vi "I2C Operation.vi"(6 "input_data":u8[](array[numeric])=[255, 255, 255, 255] format="%.0x", 7 "size":i32, 8 "Channel":u8 max=5 step=1, 9 "address":u8=123, 10 "mode":string(combo)="write", 11 "VISA":refnum<visa-resource-name>="COM3") -> (0 "VISA  2":refnum<visa-resource-name>="COM3", 1 "result":bool, 2 "message":string="no match!", 3 "Data Out":u8[](array[numeric]) format="%.0x")   [LabVIEW 2011]
panel:
  in  "write_delay":dbl=250.0
  in  "read_delay":dbl=0.1
  out "无符号字节数组":u8[](array[numeric])=[238, 0, 13, 4, 0, 161, 0, 0, 3, 4, 33, 1, 0, 0, 0, 65, 132, 128, 85, 0, 103, 0, 0, 0, 0, 0, 5, 0, 68, 69, 76, 76, 32, 32, 32, 32, 32, 32, 32, 32, 32, 32, 32, 32, 0, 60, 24, 160, 76, 53, 54, 81, 70, 48, 51, 48, 45, 83, 68, 45, 82, 32, 32, 32, 66, 32, 32, 32, 1, 0, 0, 235, 0, 0, 0, 0, 49, 54, 48, 50, 56, 48, 48, 50, 56, 32, 32, 32, 32, 32, 32, 32, 49, 54, 48, 49, 50, 56, 32, 32, 0, 0, 0, 29, 15, 16, 0, 163, 132, 0, 0, 255, 255, 255, 255, 255, 255, 255, 255, 255, 255, 255, 255, 255, 255, 255, 255, 255, 255, 255, 255, 255, 255, 255, 255, 255, 255, 255, 255, 255, 255, 255, 255, 255, 255, 255, 255, 255, 255, 255, 255, 255, 255, 255, 255, 255, 255, 255, 255, 255, 255, 255, 255, 255, 255, 255, 255, 255, 255, 255, 255, 255, 255, 255, 255, 255, 255, 255, 255, 255, 255, 255, 255, 255, 255, 255, 255, 255, 255, 255, 255, 255, 255, 255, 255, 255, 255, 255, 255, 255, 255, 255, 255, 255, 255, 255, 255, 255, 255, 255, 255, 255, 255, 255, 255, 255, 255, 255, 255, 255, 255, 255, 255, 255, 255, 255, 255, 255, 255, 255, 255, 255, 255, 255, 255, 255, 255, 255, 255, 255, 255, 255, 255, 255, 255, 255, 255, 255, 255, 255, 255, 255, 255, 255, 255, 255, 255, 255, 255, 255, 255, 255, 255, 255, 63, 255, 252, 255, 255] format="%.0x"
  out "write error":string
  out "read error":u8[](array[numeric]) format="%.0x"
  # "0"
  # "1"
  # "2"
  # "3"
  # "4"
  # "5"
  # "6"
  # "7"
  # "8"
  # "9"
  # "10"
  # "11"
  # "12"
  # "13"
  # "14"
  # "15"
  # "16"
  # "17"
  # "18"
  # "19"
  # "20"
  # "21"
  # "I2C EEPROM Opertion"
  # "10"
  # "0"
  # "5"
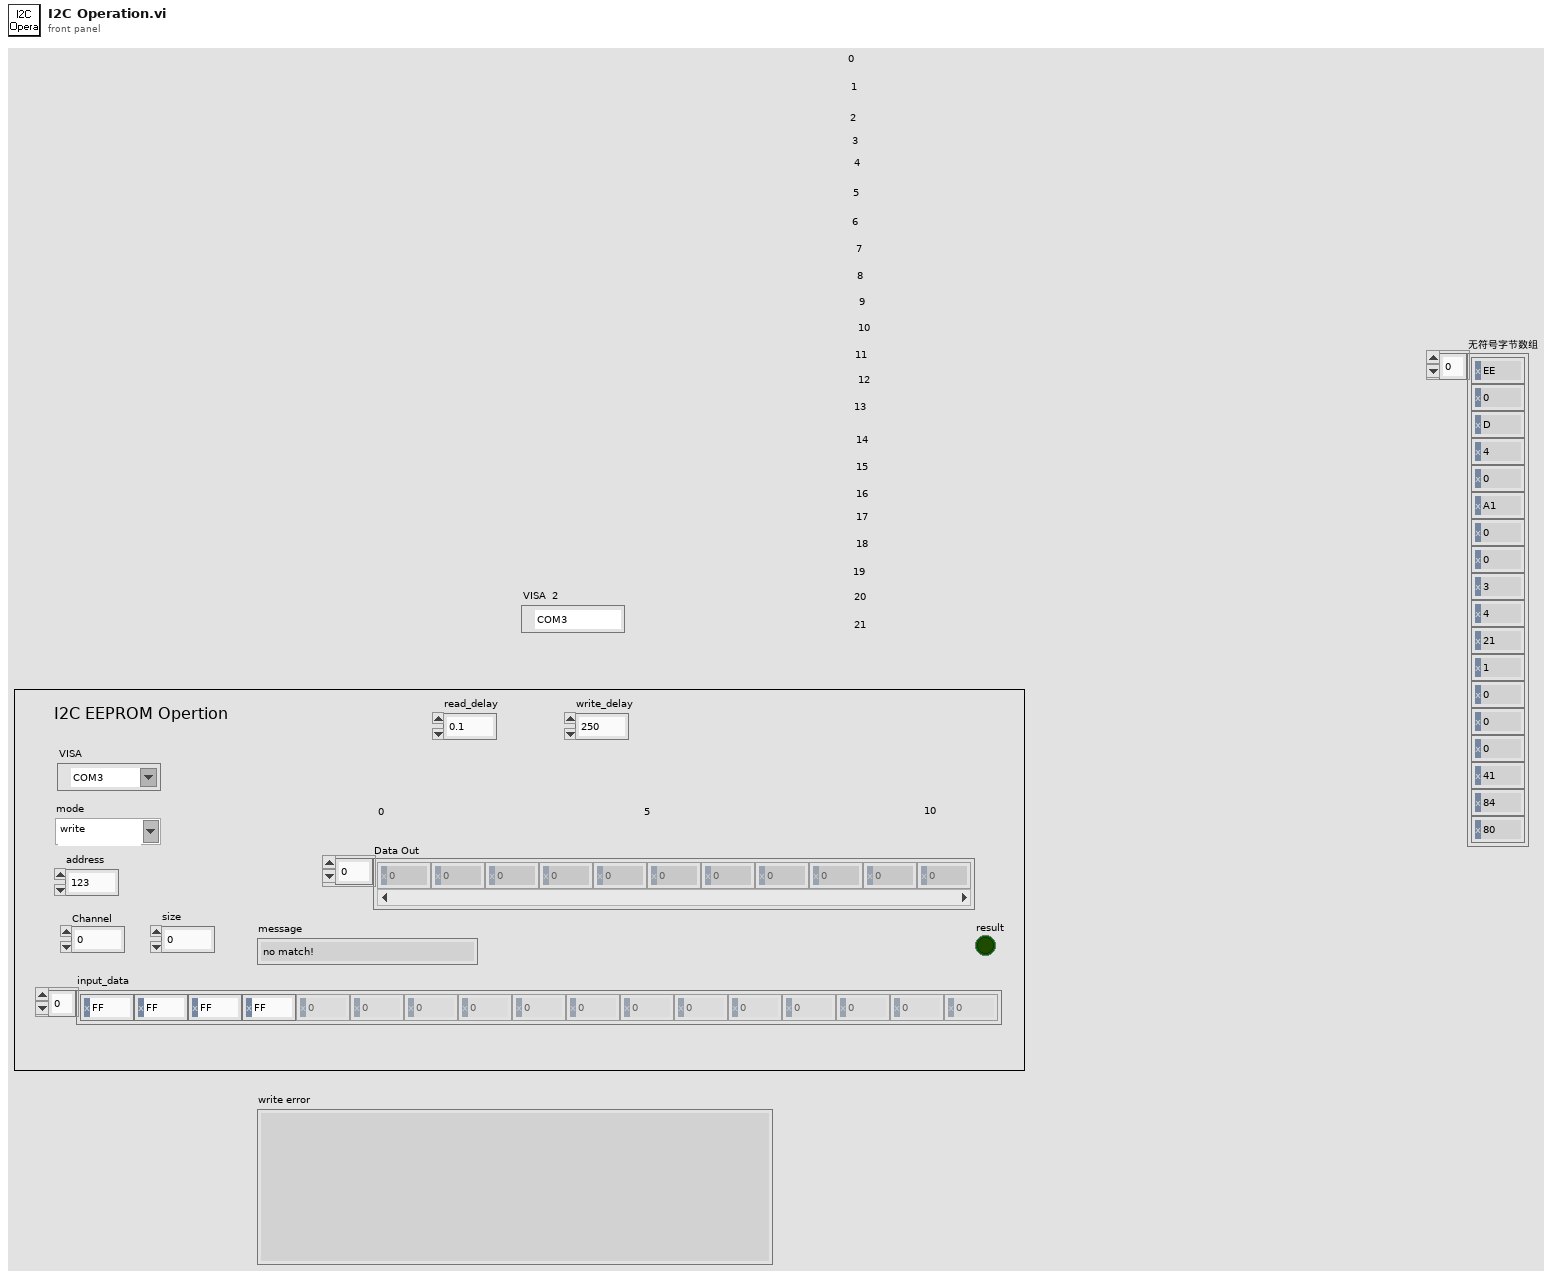
[diagram p1: front panel]
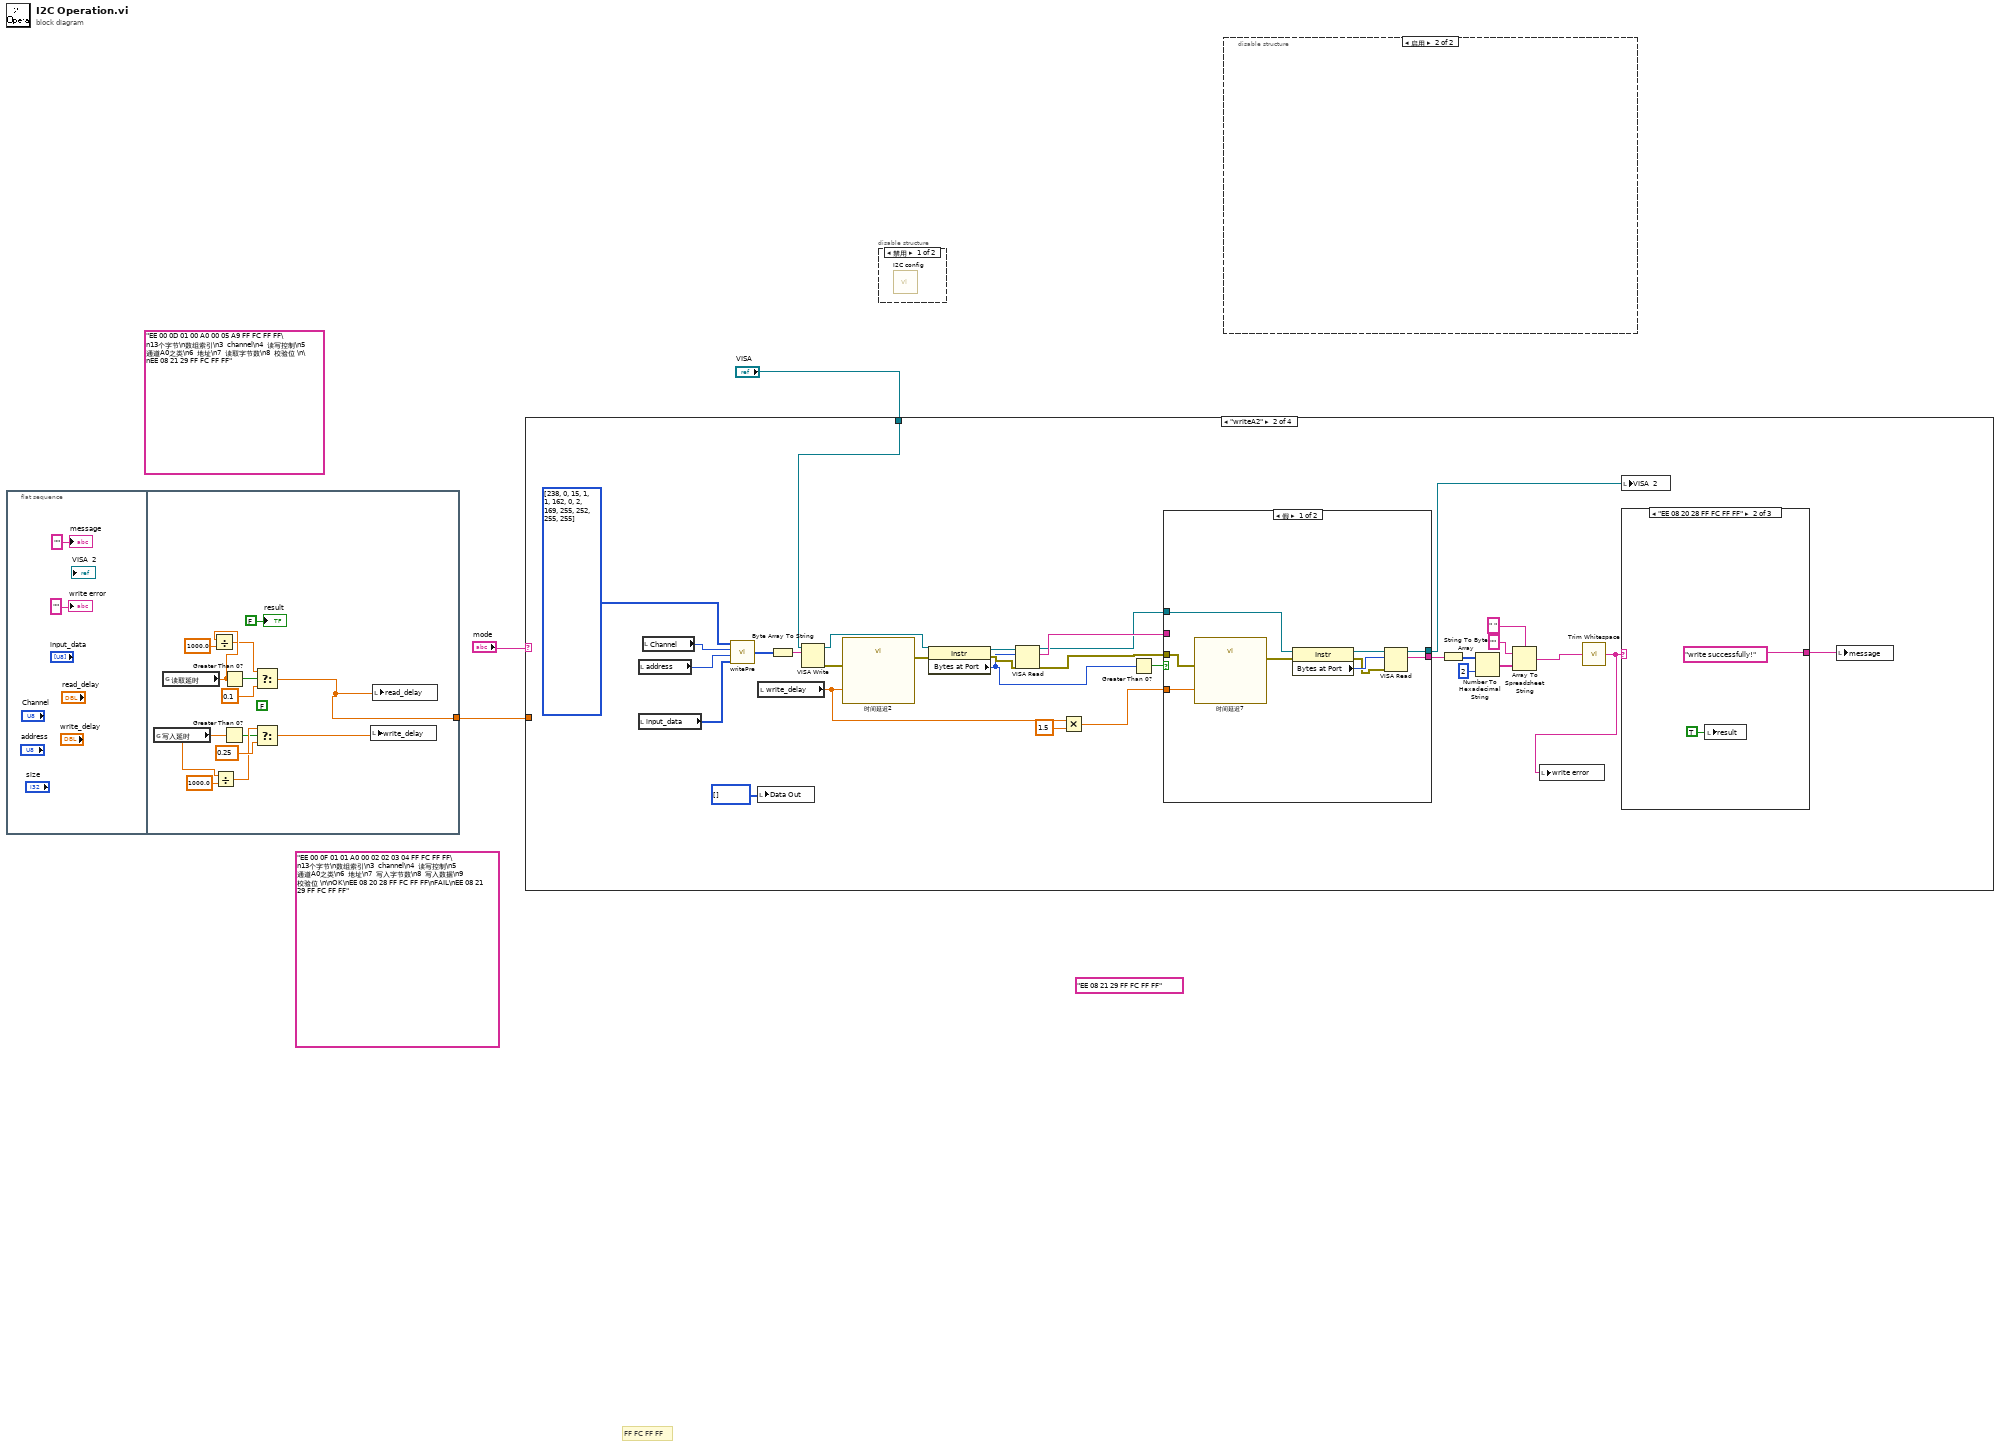
[diagram p0: block diagram]
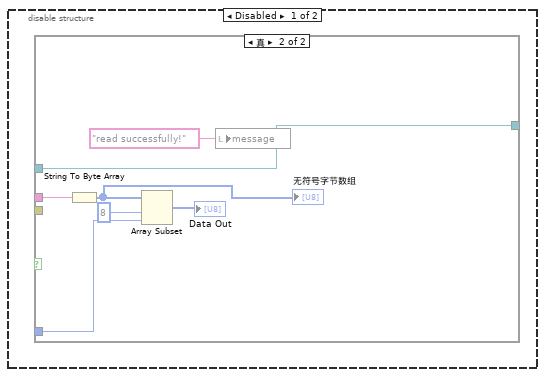
[diagram p2: hidden frame]
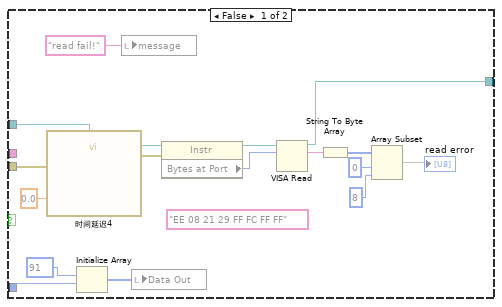
[diagram p3: hidden frame]
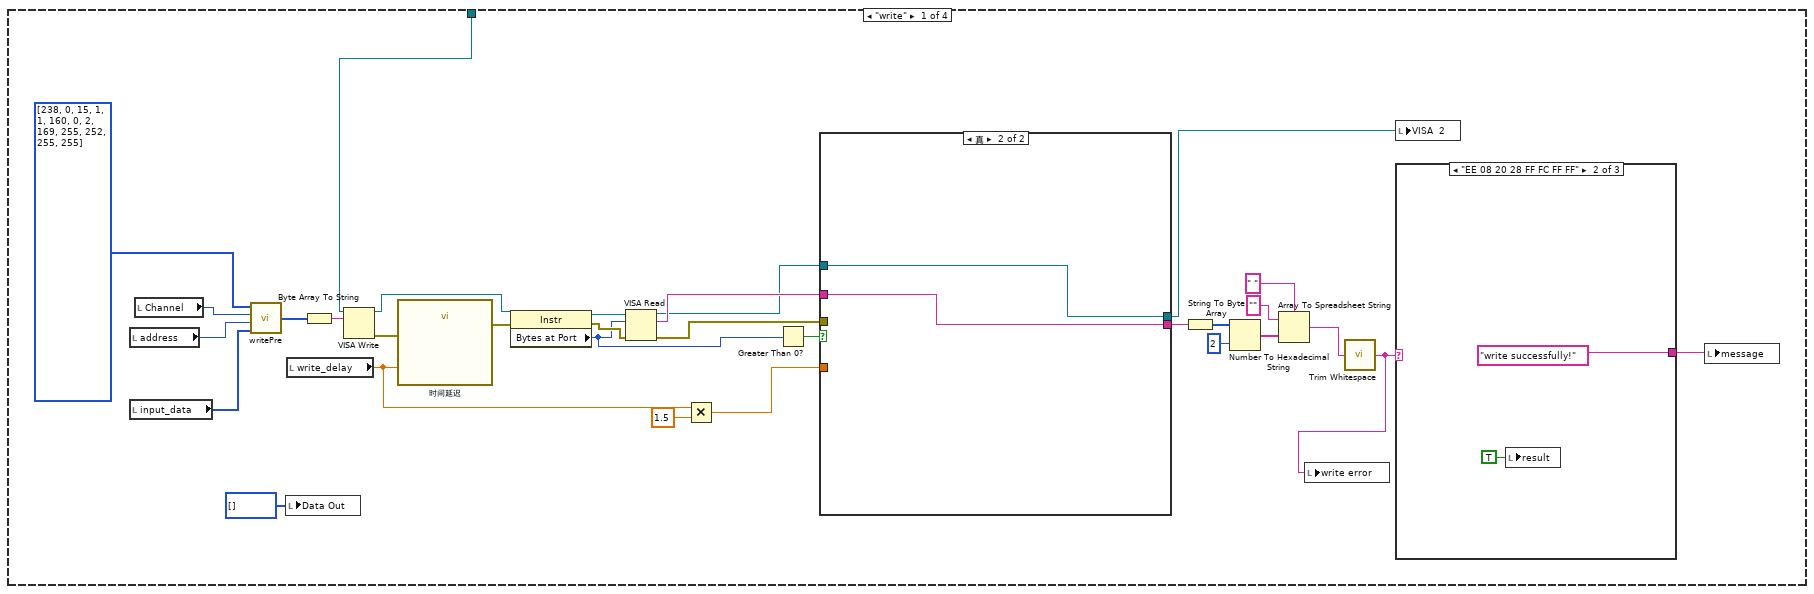
[diagram p5: hidden frame]
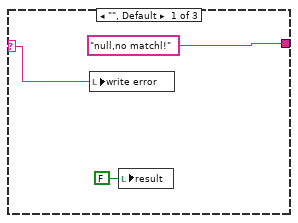
[diagram p6: hidden frame]
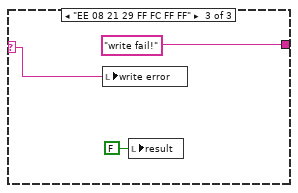
[diagram p7: hidden frame]
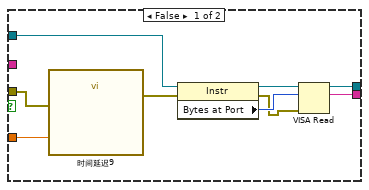
[diagram p8: hidden frame]
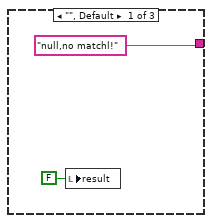
[diagram p9: hidden frame]
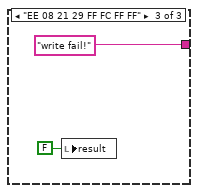
[diagram p10: hidden frame]
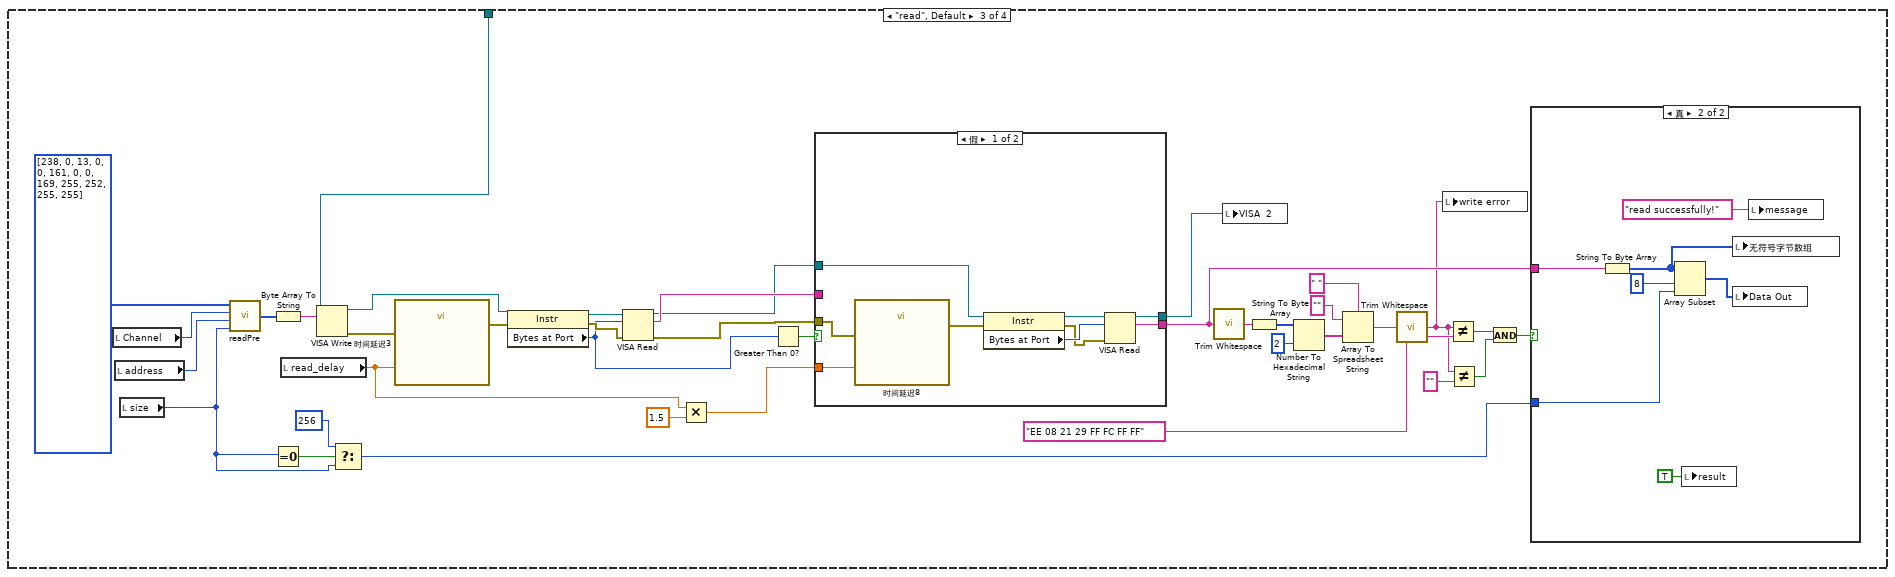
[diagram p12: hidden frame]
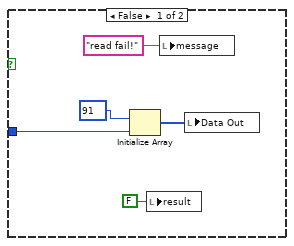
[diagram p13: hidden frame]
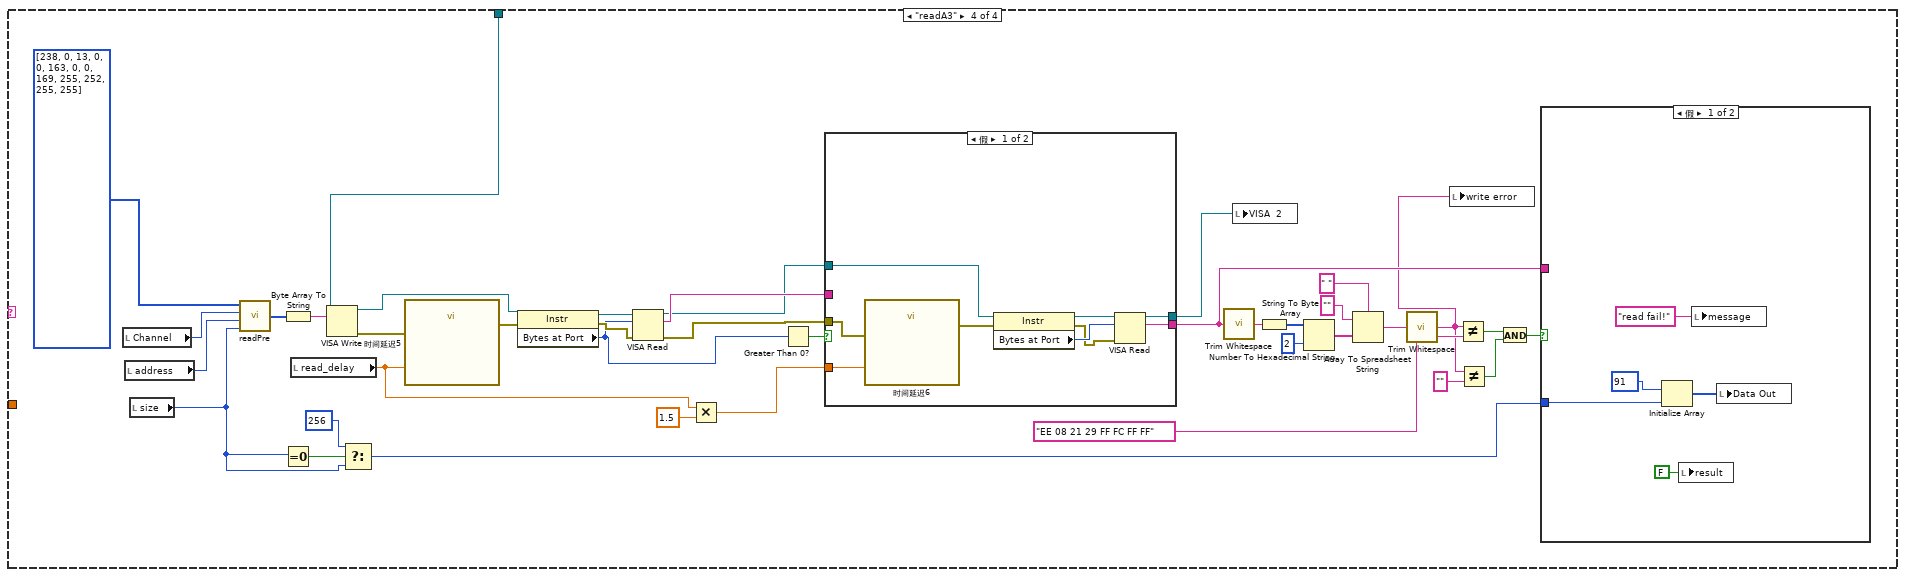
[diagram p15: hidden frame]
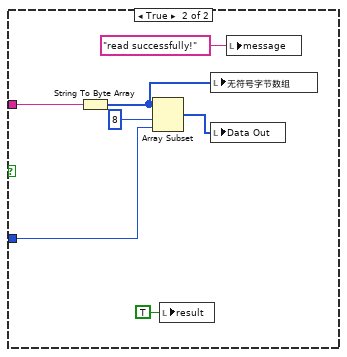
[diagram p16: hidden frame]
diagram:
  (unwired) "EE 08 21 29 FF FC FF FF"
  (unwired) "EE 00 0F 01 01 A0 00 02 02 03 04 FF FC FF FF\n13个字节\n数组索引\n3  channel\n4  读写控制\n5  通道A0之类\n6  地址\n7  写入字节数\n8  写入数据\n9  校验位 \n\nOK\nEE 08 20 28 FF FC FF FF\nFAIL\nEE 08 21 29 FF FC FF FF"
  (unwired) "EE 00 0D 01 00 A0 00 05 A9 FF FC FF FF\n13个字节\n数组索引\n3  channel\n4  读写控制\n5  通道A0之类\n6  地址\n7  读取字节数\n8  校验位 \n\nEE 08 21 29 FF FC FF FF"
  # "FF FC FF FF"
  n1 = flat-sequence {
    tunnel: [w10] -> w2
    frame #0 {
      "write error" <- "" ("write error")
      "message" <- "" ("message")
    }
    frame #1 {
      (unwired) FALSE ("s")
      n2 = global read "延时设置全局变量.vi" "写入延时"() -> (w8:dbl)
      n3 = global read "延时设置全局变量.vi" "读取延时"() -> (w12:dbl)
      n4 = Divide(x=w12, y=1000.0) -> (x/y=w11:dbl)
      n5 = Divide(x=w8, y=1000.0) -> (x/y=w9:dbl)
      n6 = Greater Than 0?(x=w8) -> (x > 0?=w6:bool)
      n7 = Greater Than 0?(x=w12) -> (x > 0?=w15:bool)
      n8 = Select(t=w9, s=w6, f=0.25) -> (s? t:f=w7:dbl)
      n9 = Select(t=w11, s=w15, f=0.1) -> (s? t:f=w10:dbl)
      n10 = local write "write_delay"(w7) -> ()
      n11 = local write "read_delay"(w10) -> ()
      "result" <- FALSE ("result")
    }
  }
  n12 = case shown="\"writeA2\"" "mode" {
    tunnel: "VISA" -> [w38 w89 w152 w213]
    tunnel: w2 -> [_ _ _ _]
    frame "write" {
      n13 = local read "address"() -> (w44:u8)
      n14 = local read "input_data"() -> (w23:u8[])
      n15 = local read "Channel"() -> (w45:u8)
      n16 = call "writePre.vi"("input_data"=w23, "address"=w44, "Channel"=w45, "order"=u8[] [238, 0, 15, 1, 1, 160, 0, 2, 169, 255, 252, 255, 255]) -> ("out"=w42:u8[])
      n17 = local write "Data Out"(u8[] [] ("Data Out")) -> ()
      n18 = local read "write_delay"() -> (w36:dbl)
      n19 = Byte Array To String(unsigned byte array=w42) -> (string=w49:string)
      n20 = VISA Write(VISA resource name=w38, write buffer=w49) -> (VISA resource name out=w39:refnum<visa-resource-name>, error out=w40:errorcluster)  [unwired: 1 in, 1 out]
      n21 = call "时间延迟"("error in (no error)"=w40, "Delay Time (s)"=w36) -> ("error out"=w47:errorcluster)  [unwired: 9 in]
      n22 = property class="Instr"(reference=w39, error in=w47) -> (reference out=w48:refnum<visa-resource-name>, error out=w46:errorcluster, "Bytes at Port"=w22:u32)
      n23 = VISA Read(VISA resource name=w48, byte count=w22, error in (no error)=w46) -> (VISA resource name out=w21:refnum<visa-resource-name>, read buffer=w26:string, error out=w20:errorcluster)  [unwired: 1 out]
      n24 = Multiply(x=w36, y=1.5) -> (x*y=w34:dbl)
      n25 = Greater Than 0?(x=w22) -> (x > 0?=w37:bool)
      n26 = case shown="真" w37 {
        tunnel: w34 -> [w66 _]
        tunnel: w20 -> [w65 _]
        tunnel: w21 -> [w64 w67]
        tunnel: [w59 w68] -> w27
        tunnel: w26 -> [_ w68]
        tunnel: [w58 w67] -> w24
        frame False {
          n27 = call "时间延迟9"("error in (no error)"=w65, "Delay Time (s)"=w66) -> ("error out"=w63:errorcluster)  [unwired: 9 in]
          n28 = property class="Instr"(reference=w64, error in=w63) -> (reference out=w62:refnum<visa-resource-name>, error out=w60:errorcluster, "Bytes at Port"=w61:u32)
          n29 = VISA Read(VISA resource name=w62, byte count=w61, error in (no error)=w60) -> (VISA resource name out=w58:refnum<visa-resource-name>, read buffer=w59:string)  [unwired: 2 out]
        }
        frame True {
        }
      }
      n30 = String To Byte Array(string=w27) -> (unsigned byte array=w33:u8[])
      n31 = Number To Hexadecimal String(1:i16 2 ("宽度(-)"), 2:w33) -> (0:w32:string[])
      n32 = Array To Spreadsheet String(delimiter (Tab)=" " ("分隔符(Tab)"), array=w32, 3:"" ("格式字符串")) -> (spreadsheet string=w29:string)
      n33 = call <vilib>:"Trim Whitespace.vi"("string"=w29) -> ("trimmed string"=w19:string)  [unwired: 1 in]
      n34 = local write "write error"(w19) -> ()
      n35 = local write "VISA  2"(w24) -> ()
      n36 = case shown="\"EE 08 20 28 FF FC FF FF\"" w19 {
        selector: w19 -> [w50 _ w55]
        tunnel: ["null,no matchl!" "write successfully!" "write fail!"] -> w25
        frame "", Default {
          n37 = local write "write error"(w50) -> ()
          n38 = local write "result"(FALSE ("result")) -> ()
        }
        frame "EE 08 20 28 FF FC FF FF" {
          n39 = local write "result"(TRUE ("result")) -> ()
        }
        frame "EE 08 21 29 FF FC FF FF" {
          n40 = local write "write error"(w55) -> ()
          n41 = local write "result"(FALSE ("result")) -> ()
        }
      }
      n42 = local write "message"(w25) -> ()
    }
    frame "writeA2" {
      n43 = local read "address"() -> (w94:u8)
      n44 = local read "input_data"() -> (w74:u8[])
      n45 = local read "Channel"() -> (w95:u8)
      n46 = call "writePre.vi"("input_data"=w74, "address"=w94, "Channel"=w95, "order"=u8[] [238, 0, 15, 1, 1, 162, 0, 2, 169, 255, 252, 255, 255]) -> ("out"=w93:u8[])
      n47 = local write "Data Out"(u8[] [] ("Data Out")) -> ()
      n48 = local read "write_delay"() -> (w87:dbl)
      n49 = Byte Array To String(unsigned byte array=w93) -> (string=w99:string)
      n50 = VISA Write(VISA resource name=w89, write buffer=w99) -> (VISA resource name out=w90:refnum<visa-resource-name>, error out=w91:errorcluster)  [unwired: 1 in, 1 out]
      n51 = call "时间延迟2"("error in (no error)"=w91, "Delay Time (s)"=w87) -> ("error out"=w97:errorcluster)  [unwired: 9 in]
      n52 = property class="Instr"(reference=w90, error in=w97) -> (reference out=w98:refnum<visa-resource-name>, error out=w96:errorcluster, "Bytes at Port"=w70:u32)
      n53 = VISA Read(VISA resource name=w98, byte count=w70, error in (no error)=w96) -> (VISA resource name out=w72:refnum<visa-resource-name>, read buffer=w77:string, error out=w71:errorcluster)  [unwired: 1 out]
      n54 = Multiply(x=w87, y=1.5) -> (x*y=w85:dbl)
      n55 = Greater Than 0?(x=w70) -> (x > 0?=w88:bool)
      n56 = case shown="假" w88 {
        tunnel: w85 -> [w114 _]
        tunnel: w71 -> [w113 _]
        tunnel: w72 -> [w112 w115]
        tunnel: [w107 w116] -> w78
        tunnel: w77 -> [_ w116]
        tunnel: [w106 w115] -> w75
        frame False {
          n57 = call "时间延迟7"("error in (no error)"=w113, "Delay Time (s)"=w114) -> ("error out"=w111:errorcluster)  [unwired: 9 in]
          n58 = property class="Instr"(reference=w112, error in=w111) -> (reference out=w110:refnum<visa-resource-name>, error out=w108:errorcluster, "Bytes at Port"=w109:u32)
          n59 = VISA Read(VISA resource name=w110, byte count=w109, error in (no error)=w108) -> (VISA resource name out=w106:refnum<visa-resource-name>, read buffer=w107:string)  [unwired: 2 out]
        }
        frame True {
        }
      }
      n60 = String To Byte Array(string=w78) -> (unsigned byte array=w84:u8[])
      n61 = Number To Hexadecimal String(1:i16 2 ("宽度(-)"), 2:w84) -> (0:w83:string[])
      n62 = Array To Spreadsheet String(delimiter (Tab)=" " ("分隔符(Tab)"), array=w83, 3:"" ("格式字符串")) -> (spreadsheet string=w80:string)
      n63 = call <vilib>:"Trim Whitespace.vi"("string"=w80) -> ("trimmed string"=w69:string)  [unwired: 1 in]
      n64 = local write "write error"(w69) -> ()
      n65 = local write "VISA  2"(w75) -> ()
      n66 = case shown="\"EE 08 20 28 FF FC FF FF\"" w69 {
        tunnel: ["null,no matchl!" "write successfully!" "write fail!"] -> w76
        frame "", Default {
          n67 = local write "result"(FALSE ("result")) -> ()
        }
        frame "EE 08 20 28 FF FC FF FF" {
          n68 = local write "result"(TRUE ("result")) -> ()
        }
        frame "EE 08 21 29 FF FC FF FF" {
          n69 = local write "result"(FALSE ("result")) -> ()
        }
      }
      n70 = local write "message"(w76) -> ()
    }
    frame "read", Default {
      n71 = local read "Channel"() -> (w123:u8)
      n72 = local read "address"() -> (w122:u8)
      n73 = local read "size"() -> (w121:i32)
      n74 = call "readPre.vi"("size"=w121, "address"=w122, "Channel"=w123, "input_order"=u8[] [238, 0, 13, 0, 0, 161, 0, 0, 169, 255, 252, 255, 255]) -> ("out"=w148:u8[])
      n75 = Byte Array To String(unsigned byte array=w148) -> (string=w154:string)
      n76 = Equal To 0?(x=w121) -> (x = 0?=w147:bool)
      n77 = local read "read_delay"() -> (w139:dbl)
      n78 = VISA Write(VISA resource name=w152, write buffer=w154) -> (VISA resource name out=w145:refnum<visa-resource-name>, error out=w144:errorcluster)  [unwired: 1 in, 1 out]
      n79 = Select(t=256, s=w147, f=w121) -> (s? t:f=w131:i32)
      n80 = call "时间延迟3"("error in (no error)"=w144, "Delay Time (s)"=w139) -> ("error out"=w151:errorcluster)  [unwired: 9 in]
      n81 = property class="Instr"(reference=w145, error in=w151) -> (reference out=w153:refnum<visa-resource-name>, error out=w150:errorcluster, "Bytes at Port"=w118:u32)
      n82 = VISA Read(VISA resource name=w153, byte count=w118, error in (no error)=w150) -> (VISA resource name out=w120:refnum<visa-resource-name>, read buffer=w140:string, error out=w119:errorcluster)  [unwired: 1 out]
      n83 = Multiply(x=w139, y=1.5) -> (x*y=w141:dbl)
      n84 = Greater Than 0?(x=w118) -> (x > 0?=w143:bool)
      n85 = case shown="假" w143 {
        tunnel: w141 -> [w175 _]
        tunnel: w119 -> [w174 _]
        tunnel: w120 -> [w173 w176]
        tunnel: [w168 w177] -> w133
        tunnel: w140 -> [_ w177]
        tunnel: [w167 w176] -> w132
        frame False {
          n86 = call "时间延迟8"("error in (no error)"=w174, "Delay Time (s)"=w175) -> ("error out"=w172:errorcluster)  [unwired: 9 in]
          n87 = property class="Instr"(reference=w173, error in=w172) -> (reference out=w171:refnum<visa-resource-name>, error out=w169:errorcluster, "Bytes at Port"=w170:u32)
          n88 = VISA Read(VISA resource name=w171, byte count=w170, error in (no error)=w169) -> (VISA resource name out=w167:refnum<visa-resource-name>, read buffer=w168:string)  [unwired: 2 out]
        }
        frame True {
        }
      }
      n89 = call <vilib>:"Trim Whitespace.vi"("string"=w133) -> ("trimmed string"=w125:string)  [unwired: 1 in]
      n90 = local write "VISA  2"(w132) -> ()
      n91 = String To Byte Array(string=w125) -> (unsigned byte array=w130:u8[])
      n92 = Number To Hexadecimal String(1:i16 2 ("宽度(-)"), 2:w130) -> (0:w129:string[])
      n93 = Array To Spreadsheet String(delimiter (Tab)=" " ("分隔符(Tab)"), array=w129, 3:"" ("格式字符串")) -> (spreadsheet string=w124:string)
      n94 = call <vilib>:"Trim Whitespace.vi"("string"=w124) -> ("trimmed string"=w117:string)  [unwired: 1 in]
      n95 = local write "write error"(w117) -> ()
      n96 = Not Equal?(x=w117, y="EE 08 21 29 FF FC FF FF") -> (x != y?=w136:bool)
      n97 = Not Equal?(x=w117, y="") -> (x != y?=w135:bool)
      n98 = And(x=w136, y=w135) -> (x .and. y?=w134:bool)
      n99 = case shown="真" w134 {
        tunnel: w133 -> [_ w165]
        tunnel: w131 -> [w156 w163]
        frame False {
          n100 = Initialize Array(u8 91, w156) -> (w157:u8[])
          n101 = local write "result"(FALSE ("result")) -> ()
          n102 = local write "message"("read fail!" ("message")) -> ()
          n103 = local write "Data Out"(w157) -> ()
        }
        frame True {
          n104 = String To Byte Array(string=w165) -> (unsigned byte array=w162:u8[])
          n105 = Array Subset(array=w162, index=8 ("索引"), length=w163) -> (w161:u8[])
          n106 = local write "result"(TRUE ("result")) -> ()
          n107 = local write "无符号字节数组"(w162) -> ()
          n108 = local write "Data Out"(w161) -> ()
          n109 = local write "message"("read successfully!" ("message")) -> ()
        }
      }
    }
    frame "readA3" {
      n110 = local read "Channel"() -> (w185:u8)
      n111 = local read "address"() -> (w184:u8)
      n112 = local read "size"() -> (w183:i32)
      n113 = call "readPre.vi"("size"=w183, "address"=w184, "Channel"=w185, "input_order"=u8[] [238, 0, 13, 0, 0, 163, 0, 0, 169, 255, 252, 255, 255]) -> ("out"=w210:u8[])
      n114 = Byte Array To String(unsigned byte array=w210) -> (string=w215:string)
      n115 = Equal To 0?(x=w183) -> (x = 0?=w209:bool)
      n116 = local read "read_delay"() -> (w201:dbl)
      n117 = VISA Write(VISA resource name=w213, write buffer=w215) -> (VISA resource name out=w207:refnum<visa-resource-name>, error out=w206:errorcluster)  [unwired: 1 in, 1 out]
      n118 = Select(t=256, s=w209, f=w183) -> (s? t:f=w193:i32)
      n119 = call "时间延迟5"("error in (no error)"=w206, "Delay Time (s)"=w201) -> ("error out"=w212:errorcluster)  [unwired: 9 in]
      n120 = property class="Instr"(reference=w207, error in=w212) -> (reference out=w214:refnum<visa-resource-name>, error out=w211:errorcluster, "Bytes at Port"=w179:u32)
      n121 = VISA Read(VISA resource name=w214, byte count=w179, error in (no error)=w211) -> (VISA resource name out=w181:refnum<visa-resource-name>, read buffer=w202:string, error out=w180:errorcluster)  [unwired: 1 out]
      n122 = Multiply(x=w201, y=1.5) -> (x*y=w203:dbl)
      n123 = Greater Than 0?(x=w179) -> (x > 0?=w205:bool)
      n124 = case shown="假" w205 {
        tunnel: w203 -> [w236 _]
        tunnel: w180 -> [w235 _]
        tunnel: w181 -> [w234 w237]
        tunnel: [w229 w238] -> w195
        tunnel: w202 -> [_ w238]
        tunnel: [w228 w237] -> w194
        frame False {
          n125 = call "时间延迟6"("error in (no error)"=w235, "Delay Time (s)"=w236) -> ("error out"=w233:errorcluster)  [unwired: 9 in]
          n126 = property class="Instr"(reference=w234, error in=w233) -> (reference out=w232:refnum<visa-resource-name>, error out=w230:errorcluster, "Bytes at Port"=w231:u32)
          n127 = VISA Read(VISA resource name=w232, byte count=w231, error in (no error)=w230) -> (VISA resource name out=w228:refnum<visa-resource-name>, read buffer=w229:string)  [unwired: 2 out]
        }
        frame True {
        }
      }
      n128 = call <vilib>:"Trim Whitespace.vi"("string"=w195) -> ("trimmed string"=w187:string)  [unwired: 1 in]
      n129 = local write "VISA  2"(w194) -> ()
      n130 = String To Byte Array(string=w187) -> (unsigned byte array=w192:u8[])
      n131 = Number To Hexadecimal String(1:i16 2 ("宽度(-)"), 2:w192) -> (0:w191:string[])
      n132 = Array To Spreadsheet String(delimiter (Tab)=" " ("分隔符(Tab)"), array=w191, 3:"" ("格式字符串")) -> (spreadsheet string=w186:string)
      n133 = call <vilib>:"Trim Whitespace.vi"("string"=w186) -> ("trimmed string"=w178:string)  [unwired: 1 in]
      n134 = local write "write error"(w178) -> ()
      n135 = Not Equal?(x=w178, y="EE 08 21 29 FF FC FF FF") -> (x != y?=w198:bool)
      n136 = Not Equal?(x=w178, y="") -> (x != y?=w197:bool)
      n137 = And(x=w198, y=w197) -> (x .and. y?=w196:bool)
      n138 = case shown="假" w196 {
        tunnel: w195 -> [_ w226]
        tunnel: w193 -> [w217 w224]
        frame False {
          n139 = Initialize Array(u8 91, w217) -> (w218:u8[])
          n140 = local write "result"(FALSE ("result")) -> ()
          n141 = local write "message"("read fail!" ("message")) -> ()
          n142 = local write "Data Out"(w218) -> ()
        }
        frame True {
          n143 = String To Byte Array(string=w226) -> (unsigned byte array=w223:u8[])
          n144 = Array Subset(array=w223, index=8 ("索引"), length=w224) -> (w222:u8[])
          n145 = local write "result"(TRUE ("result")) -> ()
          n146 = local write "无符号字节数组"(w223) -> ()
          n147 = local write "Data Out"(w222) -> ()
          n148 = local write "message"("read successfully!" ("message")) -> ()
        }
      }
    }
  }
  n149 = disable-structure shown="禁用" {
    frame Disabled {
      n150 = call "I2C config.vi"() -> ()  [unwired: 1 in, 1 out]
    }
    frame Enabled {
    }
  }
  n151 = disable-structure shown="启用" {
    frame Disabled {
      n152 = case shown="真" {
        selector: _ -> [_ _]
        tunnel: _ -> [_ w258]
        tunnel: _ -> [w250 w255]
        tunnel: _ -> [w249 _]
        tunnel: _ -> [w242 w256]
        tunnel: [w239 w255] -> _
        frame False {
          (unwired) "EE 08 21 29 FF FC FF FF"
          n153 = call "时间延迟4"("error in (no error)"=w249, "Delay Time (s)"=0.0) -> ("error out"=w252:errorcluster)  [unwired: 9 in]
          n154 = Initialize Array(u8 91, w242) -> (w240:u8[])
          n155 = local write "message"("read fail!" ("message")) -> ()
          n156 = local write "Data Out"(w240) -> ()
          n157 = property class="Instr"(reference=w250, error in=w252) -> (reference out=w253:refnum<visa-resource-name>, "Bytes at Port"=w254:u32)  [unwired: 1 out]
          n158 = VISA Read(VISA resource name=w253, byte count=w254) -> (VISA resource name out=w239:refnum<visa-resource-name>, read buffer=w244:string)  [unwired: 1 in, 2 out]
          n159 = String To Byte Array(string=w244) -> (unsigned byte array=w248:u8[])
          n160 = Array Subset(array=w248, index=0 ("索引"), length=8 ("长度")) -> (→"read error":u8[])
        }
        frame True {
          n161 = String To Byte Array(string=w258) -> (unsigned byte array=w261:u8[])
          "无符号字节数组" <- w261
          n162 = Array Subset(array=w261, index=8 ("索引"), length=w256) -> (→"Data Out":u8[])
          n163 = local write "message"("read successfully!" ("message")) -> ()
        }
      }
    }
    frame Enabled {
    }
  }
